vi "Conv_Temp.vi"(2 "Gradi Fahrenheit IN":dbl, 3 "Gradi Centigradi IN":dbl) -> (0 "Gradi Centrigradi OUT":dbl, 1 "Gradi Fahrenheit OUT":dbl)   [LabVIEW 2024]
doc: "Il programma converte i gradi Centrigradi in Fahrenheit e viceversa."
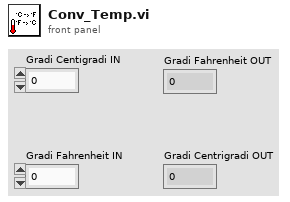
[diagram p1: front panel]
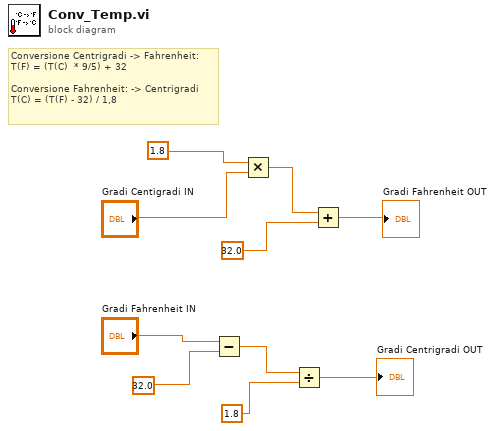
[diagram p0: block diagram]
diagram:
  # "Conversione Centrigradi -> Fahrenheit:\nT(F) = (T(C)  * 9/5) + 32\n\nConversione Fahrenheit: -> Centrigradi\nT(C) = (T(F) - 32) / 1,8"
  n1 = Subtract(x="Gradi Fahrenheit IN", y=32.0) -> (x-y=w3:dbl)
  n2 = Multiply(x=1.8, y="Gradi Centigradi IN") -> (x*y=w8:dbl)
  n3 = Divide(x=w3, y=1.8) -> (x/y=→"Gradi Centrigradi OUT":dbl)
  n4 = Add(x=w8, y=32.0) -> (x+y=→"Gradi Fahrenheit OUT":dbl)
